vi "NI_9210_Config.vi"(8 "error in":errorcluster, 11 "task in":refnum<k21>) -> (0 "error out":errorcluster, 3 "task out":refnum<k21>)   [LabVIEW 2025]
uses:
  <vilib>/DAQmx/create/channels.llb/DAQmx Create Channel (AI-Temperature-Thermocouple).vi
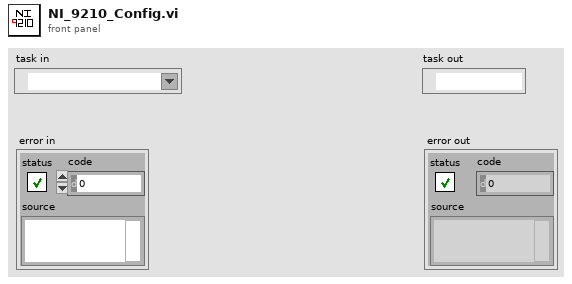
[diagram p1: front panel]
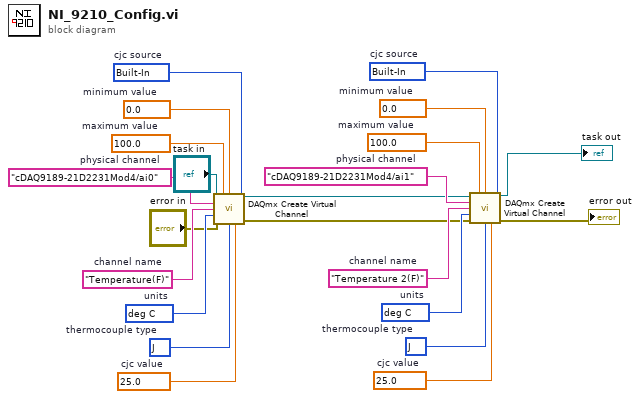
[diagram p0: block diagram]
diagram:
  w6 = 10200 items=["Built-In"=10200, "Constant Value"=10116, "Channel"=10113]  # cjc source
  w8 = 25.0  # cjc value
  w9 = 10072 items=["J"=10072, "K"=10073, "N"=10077, "R"=10082, "S"=10085, "T"=10086, "B"=10047, "E"=10055]  # thermocouple type
  w10 = 10143 items=["deg C"=10143, "deg F"=10144, "Kelvins"=10325, "deg R"=10145, "From Custom Scale"=10065]  # units
  w7 = "Temperature 2(F)"  # channel name
  w11 = 0.0  # minimum value
  w12 = 100.0  # maximum value
  w5 = "cDAQ9189-21D2231Mod4/ai1"  # physical channel
  w15 = 10200 items=["Built-In"=10200, "Constant Value"=10116, "Channel"=10113]  # cjc source
  w17 = 25.0  # cjc value
  w18 = 10072 items=["J"=10072, "K"=10073, "N"=10077, "R"=10082, "S"=10085, "T"=10086, "B"=10047, "E"=10055]  # thermocouple type
  w19 = 10143 items=["deg C"=10143, "deg F"=10144, "Kelvins"=10325, "deg R"=10145, "From Custom Scale"=10065]  # units
  w16 = "Temperature(F)"  # channel name
  w20 = 0.0  # minimum value
  w21 = 100.0  # maximum value
  w22 = "cDAQ9189-21D2231Mod4/ai0"  # physical channel
  n1 = call-poly <vilib>:"DAQmx Create Virtual Channel.vi"("task in"="task in", "maximum value"=w21, "minimum value"=w20, "physical channels"=w22, "cjc source"=w15, "name to assign"=w16, "units"=w19, "error in"="error in", "thermocouple type"=w18, "cjc value"=w17) -> ("task out"=w4:refnum<k21>, "error out"=w3:errorcluster)  [unwired: 4 in]
  n2 = call-poly <vilib>:"DAQmx Create Virtual Channel.vi"("task in"=w4, "maximum value"=w12, "minimum value"=w11, "physical channels"=w5, "cjc source"=w6, "name to assign"=w7, "units"=w10, "error in"=w3, "thermocouple type"=w9, "cjc value"=w8) -> ("task out"=→"task out":refnum<k21>, "error out"=→"error out":errorcluster)  [unwired: 4 in]
